vi "VisionAlign.vi"(11 "JoystickSpeed":dbl) -> (1 "Y":dbl, 2 "X":dbl, 3 "Z":dbl)   [LabVIEW 2018]
uses:
  <vilib>/Rock Robotics/Network Tables/NT Read Numeric Array.vi
  <vilib>/addons/control/pid/pid.llb/PID (DBL).vi
  Swerve/SwerveGlobals.vi
  <vilib>/addons/control/pid/NI_PID_pid.lvlib
panel:
  in  "AngleError":dbl=5.0
  in  "Distance PID":T1={"proportional gain (Kc)"=1.0, "integral time (Ti, min)"=0.01, "derivative time (Td, min)"=0.0} {"derivative time (Td, min)" format="%.3f"; "integral time (Ti, min)" format="%.3f"; "proportional gain (Kc)" format="%.3f"}
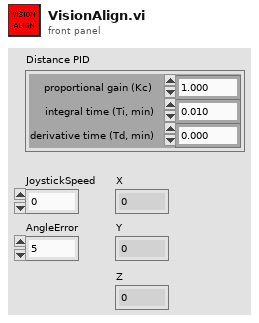
[diagram p1: front panel]
types:
  T1 = cluster{"proportional gain (Kc)":dbl, "integral time (Ti, min)":dbl, "derivative time (Td, min)":dbl}
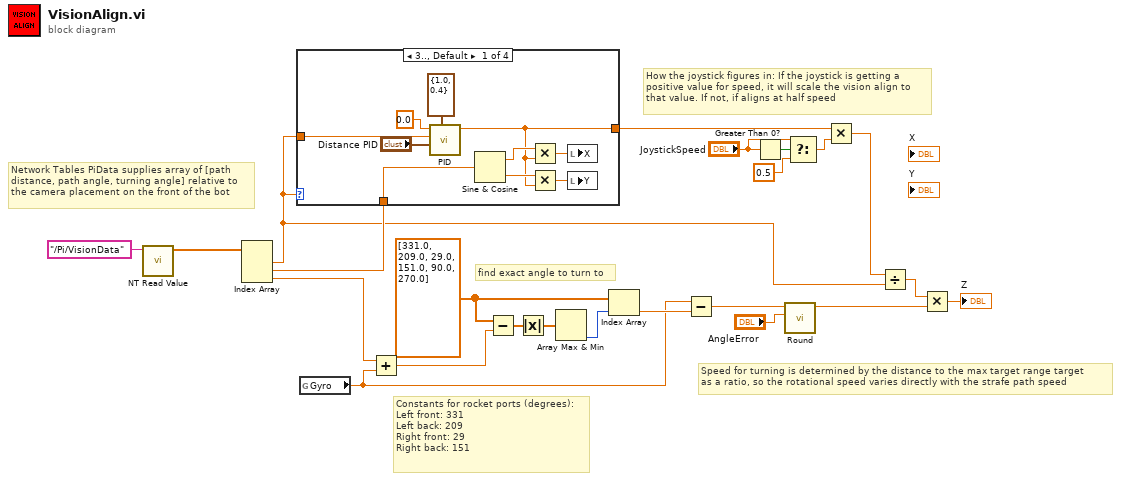
[diagram p0: block diagram]
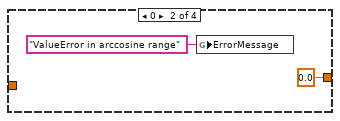
[diagram p2: hidden frame]
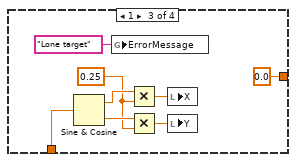
[diagram p3: hidden frame]
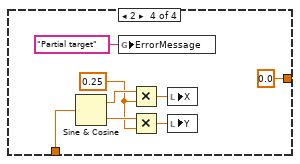
[diagram p4: hidden frame]
diagram:
  w11 = dbl[] [331.0, 209.0, 29.0, 151.0, 90.0, 270.0]
  # "find exact angle to turn to"
  # "How the joystick figures in: If the joystick is getting a\npositive value for speed, it will scale the vision align to\nthat value. If not, if aligns at half speed"
  # "Speed for turning is determined by the distance to the max target range target\nas a ratio, so the rotational speed varies directly with the strafe path speed"
  # "Constants for rocket ports (degrees):\nLeft front: 331\nLeft back: 209\nRight front: 29\nRight back: 151"
  # "Network Tables PiData supplies array of [path\ndistance, path angle, turning angle] relative to\nthe camera placement on the front of the bot"
  n1 = call-poly <vilib>:"NT Read Value.vi"("Name"="/Pi/VisionData" ("Client Name")) -> ("Numeric Array"=w22:dbl[])  [unwired: 9 in, 1 out]
  n2 = Index Array(array=w22) -> (element #1=w4:dbl, element #2=w9:dbl, element #3=w8:dbl)  [unwired: 3 in]
  n3 = case shown="3.., Default" w4 {
    tunnel: [w24 0.0 ("output") 0.0 ("output") 0.0 ("output")] -> w16
    tunnel: w4 -> [w31 _ _ _]
    tunnel: w9 -> [w25 _ w39 w47]
    frame 3.., Default {
      n4 = call-poly <vilib>:"PID.vi"("output range"=cluster{"output high":dbl, "output low":dbl} {"output high"=1.0, "output low"=0.4}, "PID gains"="Distance PID", "process variable"=w31, "setpoint"=0.0) -> ("output"=w24:dbl)  [unwired: 6 in, 1 out]
      n5 = Sine & Cosine(0:w25) -> (1:w26:dbl, 2:w27:dbl)
      n6 = Multiply(x=w26, y=w24) -> (x*y=w29:dbl)
      n7 = Multiply(x=w27, y=w24) -> (x*y=w28:dbl)
      n8 = local write "X"(w29) -> ()
      n9 = local write "Y"(w28) -> ()
    }
    frame 0 {
      n10 = global write "SwerveGlobals.vi" "ErrorMessage"("ValueError in arccosine range" ("ErrorMessage")) -> ()
    }
    frame 1 {
      w38 = 0.25 ("y")
      n11 = Sine & Cosine(0:w39) -> (1:w41:dbl, 2:w42:dbl)
      n12 = global write "SwerveGlobals.vi" "ErrorMessage"("Lone target" ("ErrorMessage")) -> ()
      n13 = Multiply(x=w41, y=w38) -> (x*y=w37:dbl)
      n14 = Multiply(x=w42, y=w38) -> (x*y=w36:dbl)
      n15 = local write "X"(w37) -> ()
      n16 = local write "Y"(w36) -> ()
    }
    frame 2 {
      w46 = 0.25 ("y")
      n17 = Sine & Cosine(0:w47) -> (1:w48:dbl, 2:w49:dbl)
      n18 = global write "SwerveGlobals.vi" "ErrorMessage"("Partial target" ("ErrorMessage")) -> ()
      n19 = Multiply(x=w48, y=w46) -> (x*y=w45:dbl)
      n20 = Multiply(x=w49, y=w46) -> (x*y=w44:dbl)
      n21 = local write "X"(w45) -> ()
      n22 = local write "Y"(w44) -> ()
    }
  }
  n23 = global read "SwerveGlobals.vi" "Gyro"() -> (w6:dbl)
  n24 = Add(x=w8, y=w6) -> (x+y=w10:dbl)
  n25 = Subtract(x=w11, y=w10) -> (x-y=w14:dbl[])
  n26 = Absolute Value(x=w14) -> (abs(x)=w13:dbl[])
  n27 = Array Max & Min(array=w13) -> (min index (indices)=w12:i32)  [unwired: 3 out]
  n28 = Index Array(array=w11, index=w12) -> (element=w7:dbl)
  n29 = Subtract(x=w6, y=w7) -> (x-y=w3:dbl)
  n30 = Greater Than 0?(x="JoystickSpeed") -> (x > 0?=w20:bool)
  n31 = call "Round.vi"("Val"="AngleError", "Step"=w3) -> ("Val'"=w2:dbl)  [unwired: 9 in]
  n32 = Select(t="JoystickSpeed", s=w20, f=0.5) -> (s? t:f=w15:dbl)
  n33 = Multiply(x=w16, y=w15) -> (x*y=w17:dbl)
  n34 = Divide(x=w17, y=w4) -> (x/y=w1:dbl)
  n35 = Multiply(x=w1, y=w2) -> (x*y=→"Z":dbl)
